vi "OpenConnectionWithDevice.vi"(8 "error in":errorcluster) -> (0 "error out":errorcluster, 2 "CCDs":refnum<class "CCD.lvclass">[](array[class]), 3 "Monos":refnum<class "Monochromator.lvclass">[](array[class]), 5 "SCDs":refnum<class "SCD.lvclass">[](array[class]))   [LabVIEW 2023, in "DeviceManager.lvlib"]
uses:
  DeviceManager.lvlib
  Classes/Mono/Monochromator.lvclass
  Classes/SCD/SCD.lvclass
  Classes/CCD/CCD.lvclass
  aa35e11d-941b-4d73-81cb-e61ed8350b73.vi
  28f67145-1fc3-4027-9ffd-6c427ba31fa2.vi
panel:
  # "Connector Pane"
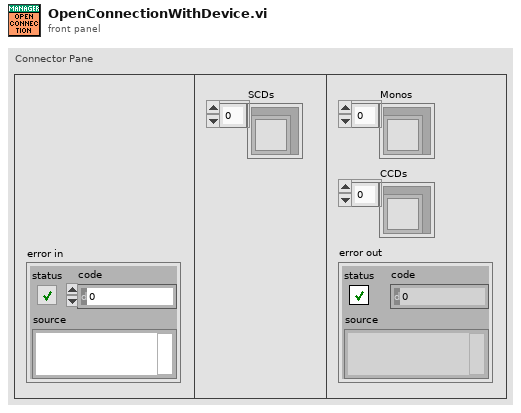
[diagram p1: front panel]
types:
  T1 = typedef "DeviceManager.lvlib/Broadcast Events--cluster.ctl" = cluster{"Module Did Init":refnum<user-event>, "Status Updated":refnum<user-event>, "Error Reported":refnum<user-event>, "Module Did Stop":refnum<user-event>, "Update Module Execution Status":refnum<user-event>}
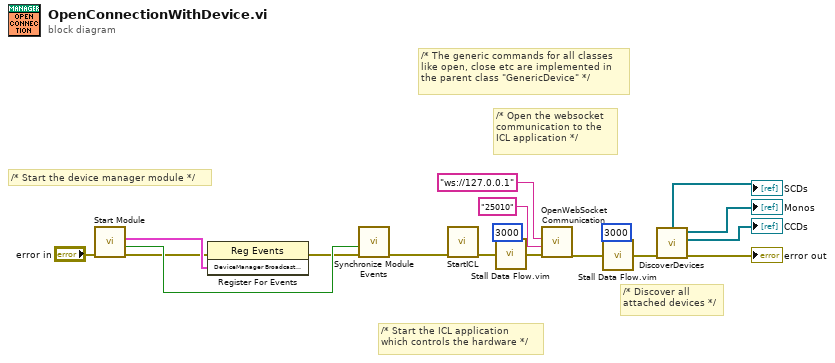
[diagram p0: block diagram]
diagram:
  # "/* The generic commands for all classes\nlike open, close etc are implemented in\nthe parent class \"GenericDevice\" */"
  # "/* Discover all\nattached devices */"
  # "/* Open the websocket\ncommunication to the \nICL application */"
  # "/* Start the ICL application\nwhich controls the hardware */"
  # "/* Start the device manager module */"
  n1 = call "Start Module.vi"("error in"="error in") -> ("error out"=w11:errorcluster, "Wait for Event Sync?"=w14:bool, "DeviceManager Broadcast Events"=w12:T1)  [unwired: 7 in, 1 out]
  n2 = register-events(error in=w11, w12) -> (error out=w13:errorcluster)  [unwired: 1 in, 1 out]
  n3 = call "Synchronize Module Events.vi"("error in"=w13, "Wait for Event Sync?"=w14) -> ("error out"=w15:errorcluster)  [unwired: 9 in]
  n4 = call "StartICL.vi"("error in"=w15) -> ("error out"=w6:errorcluster)  [unwired: 10 in]
  n5 = call "Stall Data Flow.vim"("value in"=w6, "milliseconds to wait"=u32 3000) -> ("value out"=w5:errorcluster)  [unwired: 1 out]
  n6 = call "OpenWebSocketCommunication.vi"("error in"=w5, "WS Server Port"="25010", "WS Server IP"="ws://127.0.0.1") -> ("error out"=w3:errorcluster)  [unwired: 6 in, 2 out]
  n7 = call "Stall Data Flow.vim"("value in"=w3, "milliseconds to wait"=u32 3000) -> ("value out"=w2:errorcluster)  [unwired: 1 out]
  n8 = call "DiscoverDevices.vi"("error in"=w2) -> ("error out"=→"error out":errorcluster, "CCDs"=→"CCDs":refnum<class "CCD.lvclass">[], "Monos"=→"Monos":refnum<class "Monochromator.lvclass">[], "SCDs"=→"SCDs":refnum<class "SCD.lvclass">[])  [unwired: 6 in, 1 out]
